vi "INIT_Control Panel Refs.vi"(4 "Jog":refnum<vi>, 5 "Level SP":refnum<vi>, 6 "Sim":refnum<vi>, 7 "Run Test":refnum<vi>, 8 "Flow Rate %":refnum<vi>, 9 "Level PV":refnum<vi>, 10 "Drain":refnum<vi>, 11 "Fill":refnum<vi>) -> (3 "PumpCtlRef out":T1)   [LabVIEW 2024]
uses:
  Control Definitions/Def PumpCtlRefs.ctl
panel:
  in  "Pump CtlRef In":T1
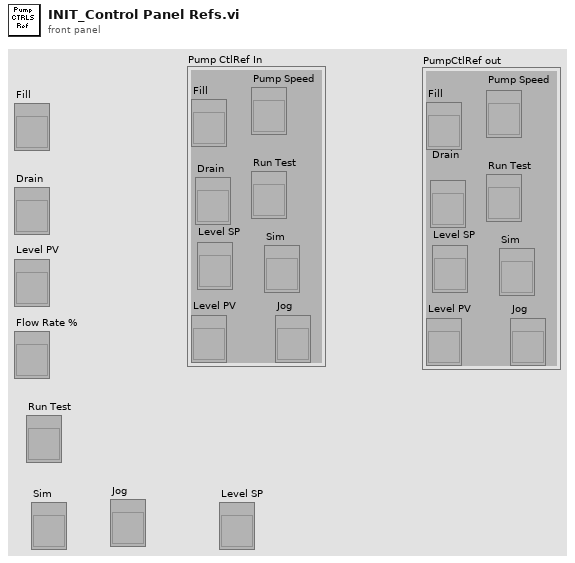
[diagram p1: front panel]
types:
  T1 = typedef "Def PumpCtlRefs.ctl" = cluster{"Fill ":refnum<vi>, "Drain":refnum<vi>, "Level PV":refnum<vi>, "Pump Speed":refnum<vi>, "Run Test":refnum<vi>, "Sim":refnum<vi>, "Jog":refnum<vi>, "Level SP":refnum<vi>}
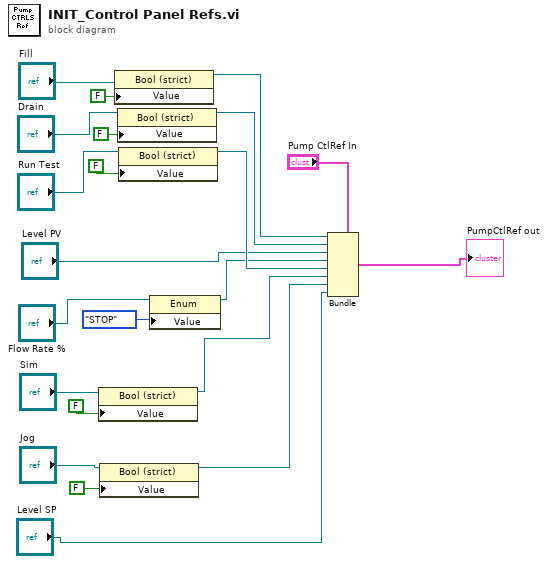
[diagram p0: block diagram]
diagram:
  n1 = property class="Bool (strict)"(reference="Sim", "Value"=FALSE) -> (reference out=w8:refnum<vi>)  [unwired: 1 in, 1 out]
  n2 = property class="Bool (strict)"(reference="Jog", "Value"=FALSE) -> (reference out=w6:refnum<vi>)  [unwired: 1 in, 1 out]
  n3 = property class="Bool (strict)"(reference="Fill", "Value"=FALSE) -> (reference out=w20:refnum<vi>)  [unwired: 1 in, 1 out]
  n4 = property class="Bool (strict)"(reference="Drain", "Value"=FALSE) -> (reference out=w16:refnum<vi>)  [unwired: 1 in, 1 out]
  n5 = property class="Bool (strict)"(reference="Run Test", "Value"=FALSE) -> (reference out=w13:refnum<vi>)  [unwired: 1 in, 1 out]
  n6 = property class="Enum"(reference="Flow Rate %", "Value"=enum16{"FAST", "SLOW", "CREEP", "STOP"}."STOP" ("Pump Speed")) -> (reference out=w11:refnum<vi>)  [unwired: 1 in, 1 out]
  n7 = Bundle(cluster="Pump CtlRef In", "Fill"=w20, "Drain"=w16, "Level PV"="Level PV", "Pump Speed"=w11, "Run Test"=w13, "Sim"=w8, "Jog"=w6, "Level SP"="Level SP") -> (→"PumpCtlRef out":T1)
